vi "MTM2_getSample_tangentEncoderPositions.vi"(8 "error in (no error)":errorcluster, 11 "tangentEncoderPositions_Ctl":T1={"private_rcvStamp"=0.0, "position[6]"=[0.0, 0.0, 0.0, 0.0, 0.0, 0.0]}) -> (0 "error out":errorcluster, 2 "function return":i32, 3 "tangentEncoderPositions_Ctl out":T1)   [LabVIEW 2018, in "SALLV_MTM2.lvlib"]
doc: "int MTM2_shm_getSample_tangentEncoderPositionsLV(MTM2_tangentEncoderPositionsLV *tangentEncoderPositions_Ctl );"
uses:
  DataTypes/tangentEncoderPositions.ctl
  SALLV_MTM2.lvlib
  SALLV_MTM2.so
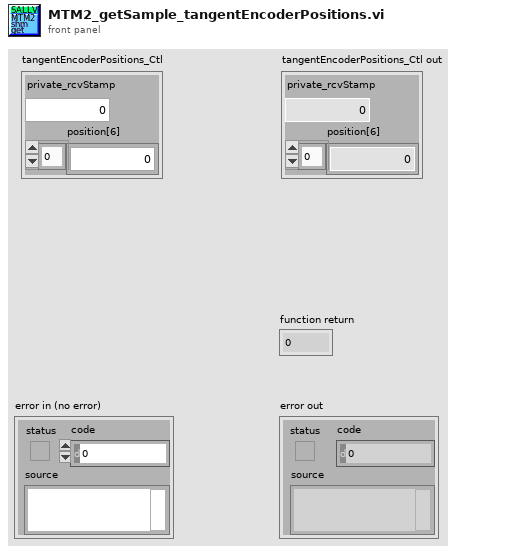
[diagram p1: front panel]
types:
  T1 = typedef "SALLV_MTM2.lvlib/tangentEncoderPositions.ctl" = cluster{"private_rcvStamp":dbl, "position[6]":dbl[]}
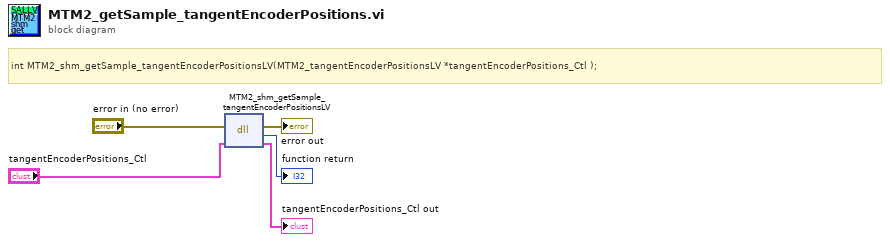
[diagram p0: block diagram]
diagram:
  # "int MTM2_shm_getSample_tangentEncoderPositionsLV(MTM2_tangentEncoderPositionsLV *tangentEncoderPositions_Ctl );"
  n1 = dll-call lib="home/ttsai/Documents/salTestLabViewApi/SALLV_MTM2/SALLV_MTM2.*" fn="MTM2_shm_getSample_tangentEncoderPositionsLV"(error in="error in (no error)", "tangentEncoderPositions_Ctl"="tangentEncoderPositions_Ctl") -> (error out=→"error out":errorcluster, →"function return":i32, "tangentEncoderPositions_Ctl"=→"tangentEncoderPositions_Ctl out":T1)  [unwired: 2 in, 1 out]
